vi "PH_Beamline.set GUI Refs.vi"(0 "i ref in":refnum<vi>, 1 "Class":string, 2 "PH Beamline GUI Refs":T3, 3 "PH_BL-Master GUI Refs":T2, 4 "System Information GUI Refs":T1, 5 "error in (no error)":errorcluster) -> (14 "i ref out":refnum<vi>, 19 "error out":errorcluster)   [LabVIEW 2014, in "PH_Beamline.lvlib"]
uses:
  PH_Beamline.lvlib
  PH_Beamline.GUI Refs.ctl
  PH_BL-Master/PH_BL-Master.GUI Refs.ctl
  PH_SystemInformation/PH_SystemInformation.GUI Refs.ctl
  PH_BL-Master/PH_BL-Master.lvlib
  PH_SystemInformation/PH_SystemInformation.lvlib
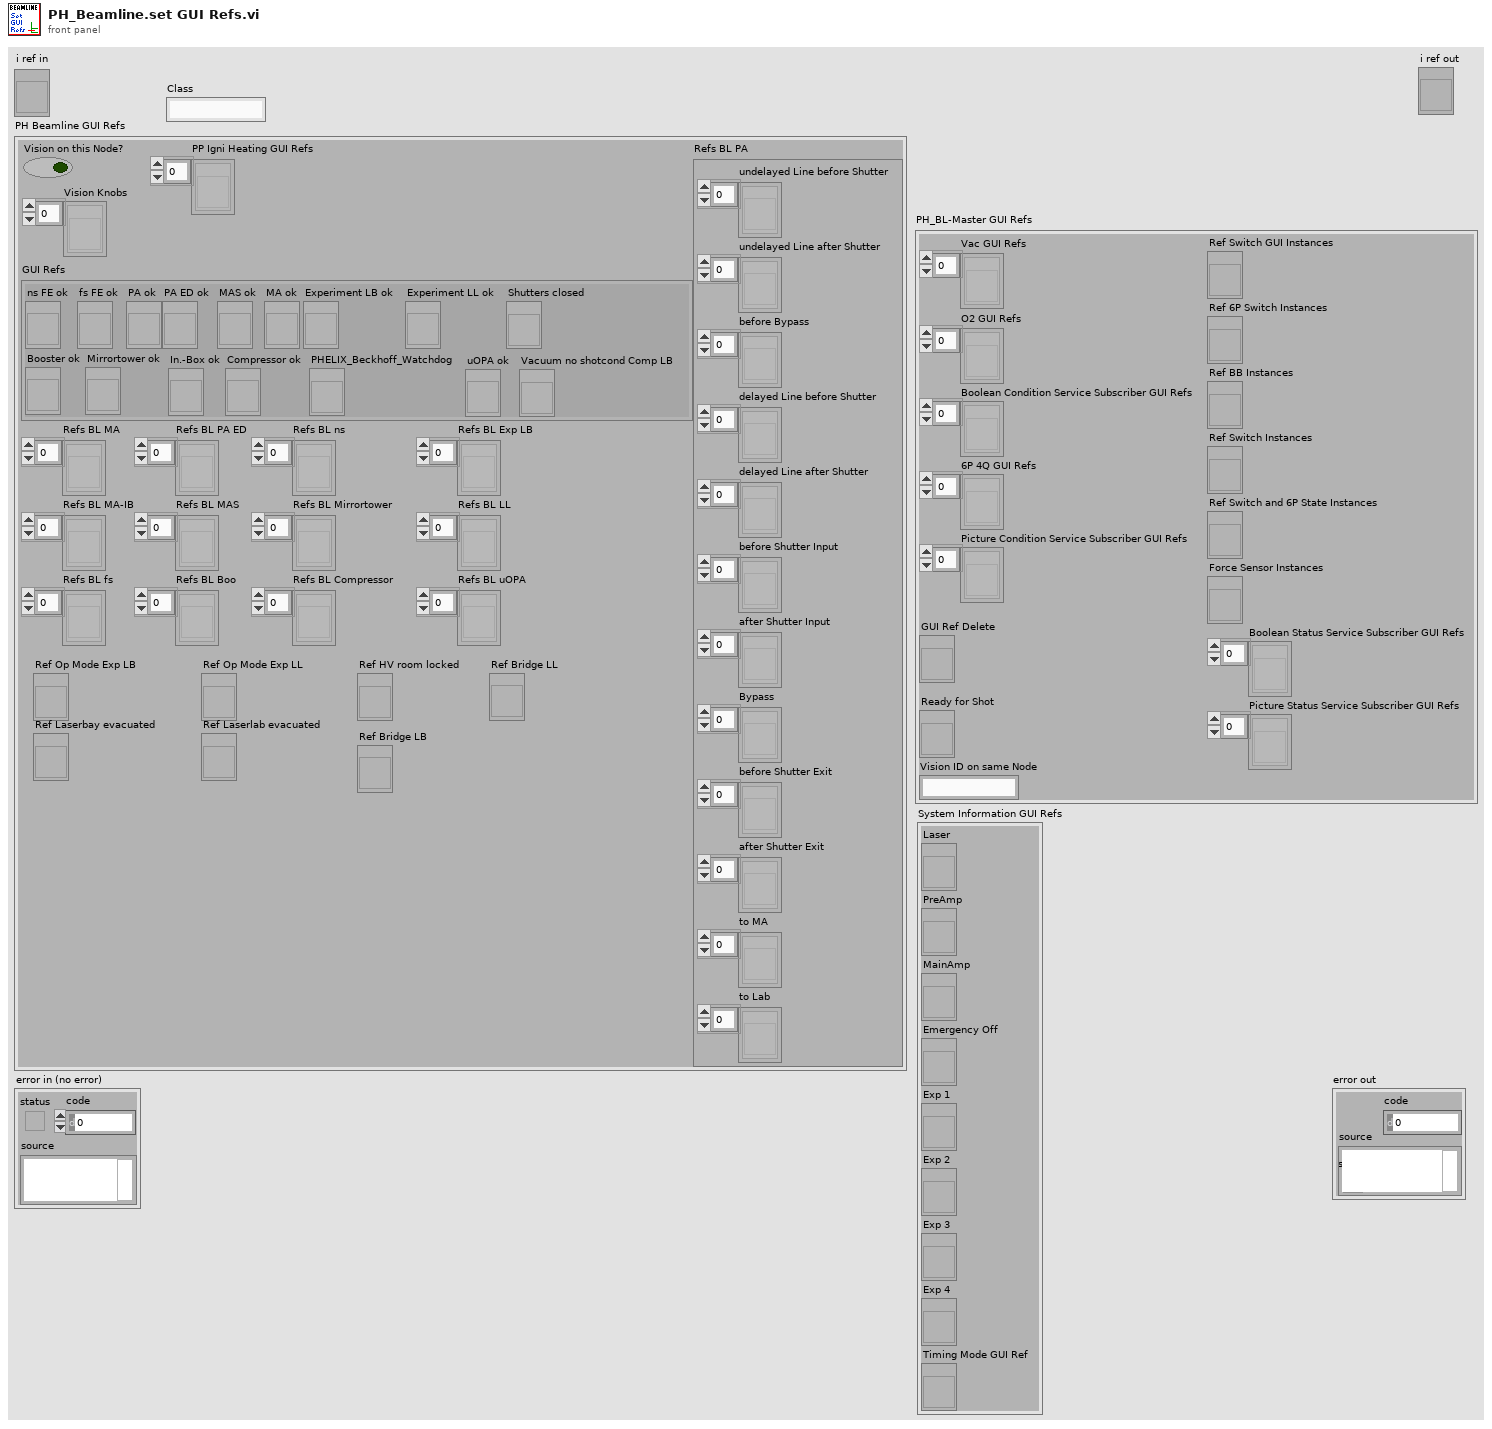
[diagram p1: front panel]
types:
  T1 = typedef "PH_SystemInformation.lvlib/PH_SystemInformation.GUI Refs.ctl" = cluster{"Laser":refnum<vi>, "PreAmp":refnum<vi>, "MainAmp":refnum<vi>, "Emergency Off":refnum<vi>, "Exp 1":refnum<vi>, "Exp 2":refnum<vi>, "Exp 3":refnum<vi>, "Exp 4":refnum<vi>, "Timing Mode GUI Ref":refnum<vi>}
  T2 = typedef "PH_BL-Master.lvlib/PH_BL-Master.GUI Refs.ctl" = cluster{"Vac GUI Refs":refnum<vi>[], "O2 GUI Refs":refnum<vi>[], "Ready for Shot":refnum<vi>, "Boolean Condition Service Subscriber GUI Refs":refnum<vi>[], "Vision ID on same Node":string, "Picture Condition Service Subscriber GUI Refs":refnum<vi>[], "6P 4Q GUI Refs":refnum<vi>[], "Ref Switch GUI Instances":refnum<vi>, "Ref 6P Switch Instances":refnum<vi>, "Ref BB Instances":refnum<vi>, "Ref Switch Instances":refnum<vi>, "Ref Switch and 6P State Instances":refnum<vi>, "Boolean Status Service Subscriber GUI Refs":refnum<vi>[], "Picture Status Service Subscriber GUI Refs":refnum<vi>[], "Force Sensor Instances":refnum<vi>, "GUI Ref Delete":refnum<vi>}
  T3 = typedef "PH_Beamline.lvlib/PH_Beamline.GUI Refs.ctl" = cluster{"Vision on this Node?":bool, "Vision Knobs":refnum<vi>[], "GUI Refs":cluster{"PA ok":refnum<vi>, "MA ok":refnum<vi>, "fs FE ok":refnum<vi>, "ns FE ok":refnum<vi>, "PA ED ok":refnum<vi>, "MAS ok":refnum<vi>, "Booster ok":refnum<vi>, "Mirrortower ok":refnum<vi>, "In.-Box ok":refnum<vi>, "Compressor ok":refnum<vi>, "Experiment LB ok":refnum<vi>, "Experiment LL ok":refnum<vi>, "PHELIX_Beckhoff_Watchdog":refnum<vi>, "Shutters closed":refnum<vi>, "uOPA ok":refnum<vi>, "Vacuum no shotcond Comp LB":refnum<vi>}, "PP Igni Heating GUI Refs":refnum<vi>[], "Refs BL PA":cluster{"undelayed Line before Shutter":refnum<vi>[], "undelayed Line after Shutter":refnum<vi>[], "before Bypass":refnum<vi>[], "delayed Line before Shutter":refnum<vi>[], "delayed Line after Shutter":refnum<vi>[], "before Shutter Input":refnum<vi>[], "after Shutter Input":refnum<vi>[], "Bypass":refnum<vi>[], "before Shutter Exit":refnum<vi>[], "after Shutter Exit":refnum<vi>[], "to MA":refnum<vi>[], "to Lab":refnum<vi>[]}, "Refs BL MA":refnum<vi>[], "Refs BL MA-IB":refnum<vi>[], "Refs BL fs":refnum<vi>[], "Refs BL PA ED":refnum<vi>[], "Refs BL MAS":refnum<vi>[], "Refs BL Boo":refnum<vi>[], "Refs BL ns":refnum<vi>[], "Refs BL Mirrortower":refnum<vi>[], "Refs BL Compressor":refnum<vi>[], "Refs BL Exp LB":refnum<vi>[], "Refs BL LL":refnum<vi>[], "Refs BL uOPA":refnum<vi>[], "Ref Op Mode Exp LB":refnum<vi>, "Ref Laserbay evacuated":refnum<vi>, "Ref Op Mode Exp LL":refnum<vi>, "Ref Laserlab evacuated":refnum<vi>, "Ref HV room locked":refnum<vi>, "Ref Bridge LB":refnum<vi>, "Ref Bridge LL":refnum<vi>}
  T4 = cluster{"undelayed Line before Shutter":refnum<vi>[], "undelayed Line after Shutter":refnum<vi>[], "before Bypass":refnum<vi>[], "delayed Line before Shutter":refnum<vi>[], "delayed Line after Shutter":refnum<vi>[], "before Shutter Input":refnum<vi>[], "after Shutter Input":refnum<vi>[], "Bypass":refnum<vi>[], "before Shutter Exit":refnum<vi>[], "after Shutter Exit":refnum<vi>[], "to MA":refnum<vi>[], "to Lab":refnum<vi>[]}
  T5 = cluster{"PA ok":refnum<vi>, "MA ok":refnum<vi>, "fs FE ok":refnum<vi>, "ns FE ok":refnum<vi>, "PA ED ok":refnum<vi>, "MAS ok":refnum<vi>, "Booster ok":refnum<vi>, "Mirrortower ok":refnum<vi>, "In.-Box ok":refnum<vi>, "Compressor ok":refnum<vi>, "Experiment LB ok":refnum<vi>, "Experiment LL ok":refnum<vi>, "PHELIX_Beckhoff_Watchdog":refnum<vi>, "Shutters closed":refnum<vi>, "uOPA ok":refnum<vi>, "Vacuum no shotcond Comp LB":refnum<vi>}
  T6 = typedef "PH_Beamline.lvlib/PH_Beamline.i attribute.ctl" = cluster{"GUI Refs":cluster{"PA ok":refnum<vi>, "MA ok":refnum<vi>, "fs FE ok":refnum<vi>, "ns FE ok":refnum<vi>, "PA ED ok":refnum<vi>, "MAS ok":refnum<vi>, "Booster ok":refnum<vi>, "Mirrortower ok":refnum<vi>, "In.-Box ok":refnum<vi>, "Compressor ok":refnum<vi>, "Experiment LB ok":refnum<vi>, "Experiment LL ok":refnum<vi>, "PHELIX_Beckhoff_Watchdog":refnum<vi>, "Shutters closed":refnum<vi>, "uOPA ok":refnum<vi>, "Vacuum no shotcond Comp LB":refnum<vi>}, "Refs BL MA":refnum<vi>[], "Refs BL MA-IB":refnum<vi>[], "Refs BL fs":refnum<vi>[], "Refs BL PA ED":refnum<vi>[], "Refs BL MAS":refnum<vi>[], "Refs BL Boo":refnum<vi>[], "Refs BL ns":refnum<vi>[], "Refs BL Mirrortower":refnum<vi>[], "Refs BL Compressor":refnum<vi>[], "Refs BL Exp LB":refnum<vi>[], "Radiation Safety":cluster{"Exp Laserbay":cluster{"Ref Op Mode":refnum<vi>, "Ref Laserbay evacuated":refnum<vi>, "Tagname LB evacuated":string, "Shot Mode":T7, "Laserbay evacuated?":i32, "Tagname HV room locked":string, "HV room locked?":i32, "Ref HV room locked":refnum<vi>, "Tagname bridged?":string, "Ref Bridge":refnum<vi>, "I<1E18W/cm²":bool}, "Exp Laserlab":cluster{"Ref Op Mode":refnum<vi>, "Ref Laserlab evacuated":refnum<vi>, "Tagname LL evacuated":string, "Shot Mode":T7, "Laserlab evacuated?":i32, "Tagname bridged?":string, "Ref Bridge":refnum<vi>, "I<1E18W/cm²":bool}}, "Refs BL LL":refnum<vi>[], "PP Igni Heating GUI Refs":refnum<vi>[], "PP Igni Heating Tagnames ":string[], "Refs BL PA":cluster{"undelayed Line before Shutter":refnum<vi>[], "undelayed Line after Shutter":refnum<vi>[], "before Bypass":refnum<vi>[], "delayed Line before Shutter":refnum<vi>[], "delayed Line after Shutter":refnum<vi>[], "before Shutter Input":refnum<vi>[], "after Shutter Input":refnum<vi>[], "Bypass":refnum<vi>[], "before Shutter Exit":refnum<vi>[], "after Shutter Exit":refnum<vi>[], "to MA":refnum<vi>[], "to Lab":refnum<vi>[]}, "BL":cluster{"YLF_BL_Status":i32, "fs_BL_Status":i32, "fs_YLF_BL_Status":i32, "ns_BL_Status":i32, "PA_Input_BL_Status":i32, "PA_UnDelay_BL_Status":i32, "PA_Delay_BL_Status":i32, "PA_BL_Status":i32, "PA_Bypass_BL_Status":i32, "PA_Exit_BL_Status":i32, "PA_LL_BL_Status":i32, "LL_BL_Status":i32, "PA_MA_BL_Status":i32, "MA_Exit_BL_Status":i32, "MA_Z6_BL_Status":i32, "Z6_BL_Status":i32, "MA_LB_BL_Status":i32, "LB_TB2_BL_Status":i32, "PA_before_Bypass_BL_Status":i32, "LB_TB3_BL_Status":i32}, "State Subsystems":cluster{"PA":bool, "MA":bool, "ns FE":bool, "fs FE":bool, "PA ED":bool, "In.-Box":bool, "MAS":bool, "Booster":bool, "Mirrortower":bool, "Compressor":bool, "Experiment LB":bool, "Experiment LL":bool, "uOPA":bool}, "Status Subscriber Information":T8, "Refs BL uOPA":refnum<vi>[], "PA_Input_2_Beam_6PWpGUI not linked?":bool, "PA_Input_Delay_6PGUI not linked?":bool, "Settings":T11}
  T7 = typedef "PH_Beamline.lvlib/PH_Beamline.Operation Mode.ctl" = i32
  T8 = typedef "PH_Beamline.lvlib/PH_Beamline.Status Subscriber Information.ctl" = cluster{"fs Swich YLF":T9, "fs Exit Shutter":T9, "ns Exit Shutter":T9, "PA Input Shutter":T9, "PA PC WP":T9, "PA PC WP 2":T9, "PA Bypass In":T9, "PA Bypass Out":T9, "PA CH 1":T9, "PA delayed":T9, "PA non delayed":T9, "PA Exit Shutter":T9, "PA Switch Lab":T9, "PA Bridge CH Input MA":T9, "MA Diffusor IB":T9, "MA IB Ready":T9, "MA CH 1":T9, "MA CH 2":T9, "MA CH 3":T9, "MA CH 4":T9, "MA Shutter Align Cam":T9, "MA Position MM5":T9, "Calorimeter Switch":T9, "BL Z6 CH 9":T9, "BL Z6 Beamdump":T9, "BL Z6 Shutter":T9, "COS Sensitivity Switch":T9, "Exp LB Shutter":T9, "Exp LB TB 2":T9, "Exp LB TB 3":T9, "PA LL Input CH":T9, "PA LL Output CH":T9, "LL Comp Input Shutter":T9, "LL Comp Output Shutter":T9, "LL Comp FF Shutter":T9, "Exp LL Shutter":T9, "MA IM In IB":T9, "MA IM Out IB":T9, "MA DB In IB":T9, "MA DB Out IB":T9, "Exp LB Shutter Interlock":T9, "Exp LL Shutter Interlock":T9, "MM1 Force Sensor":T9}
  T9 = typedef "PH_BL-Master.lvlib/PH_BL-Master.Status Subscriber Information.ctl" = cluster{"Index of element":i32, "Attributeset":T10}
  T10 = typedef "PH_BL-Master.lvlib/PH_BL-Master.Attribute Set.ctl" = enum16{"Boolean Status Service Subscriber", "Picture Status Service Subscriber"}
  T11 = typedef "PH_Beamline_Chief.lvlib/PH_Beamline_Chief.Settings.ctl" = cluster{"PA Doublepass Mode":bool, "Compressor Vaccuum LB not relevant":bool, "Windowshutter TB2 not relevant":bool, "Windowshutter TB3 not relevant":bool}
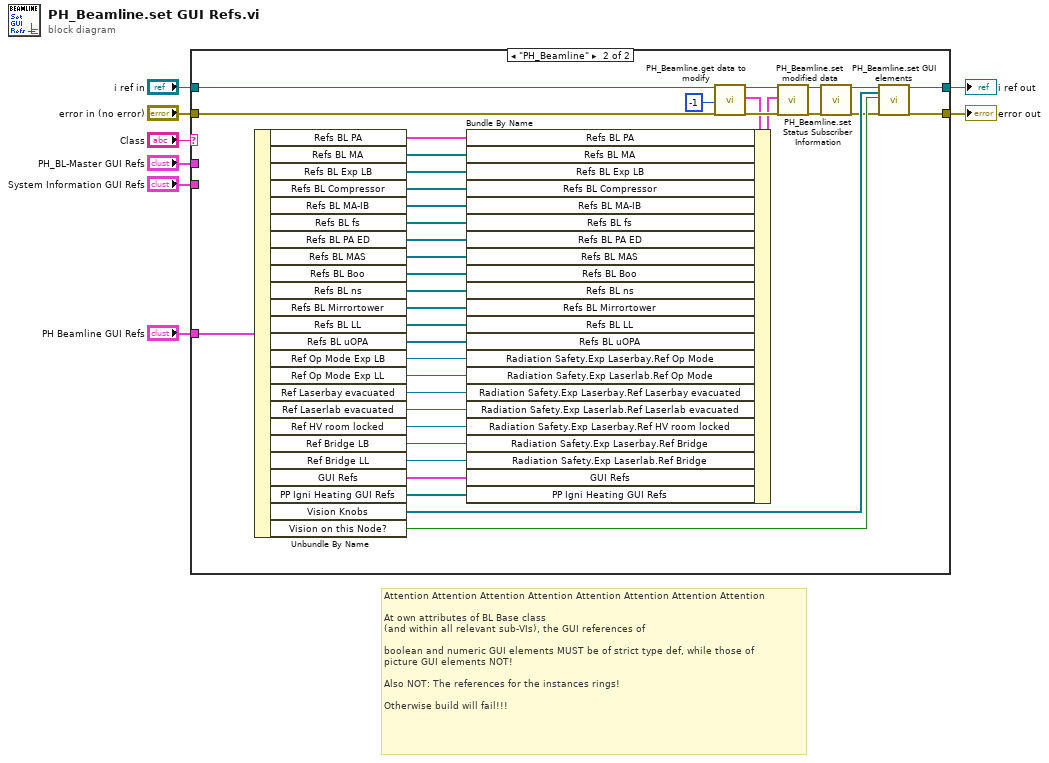
[diagram p0: block diagram]
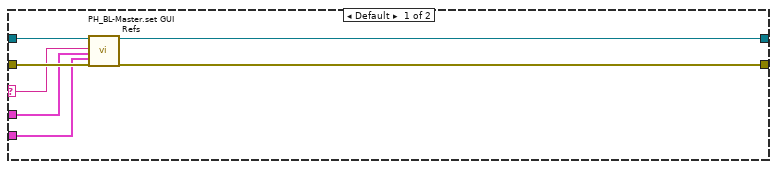
[diagram p2: hidden frame]
diagram:
  # "Attention Attention Attention Attention Attention Attention Attention Attention\n\nAt own attributes of BL Base class \n(and within all relevant sub-VIs), the GUI references of\n\nboolean and numeric GUI elements MUST be of strict type def, while those of\npicture GUI elements NOT!\n\nAlso NOT: The references for the instances rings!\n\nOtherwise build will fail!!!"
  n1 = case shown="\"PH_Beamline\"" "Class" {
    selector: "Class" -> [w11 _]
    tunnel: "i ref in" -> [w15 w53]
    tunnel: "error in (no error)" -> [w14 w52]
    tunnel: [w13 w51] -> w6
    tunnel: [w12 w50] -> w5
    tunnel: "PH Beamline GUI Refs" -> [_ w49]
    tunnel: "PH_BL-Master GUI Refs" -> [w10 _]
    tunnel: "System Information GUI Refs" -> [w9 _]
    frame Default {
      n2 = call "PH_BL-Master.set GUI Refs.vi"("i ref in"=w15, "Class"=w11, "PH_BL-Master GUI Refs"=w10, "System Information GUI Refs"=w9, "error in"=w14) -> ("i ref out"=w13:refnum<vi>, "error out"=w12:errorcluster)  [unwired: 13 in]
    }
    frame "PH_Beamline" {
      n3 = Unbundle By Name(w49) -> ("Refs BL PA"=w25:T4, "Refs BL MA"=w26:refnum<vi>[], "Refs BL Exp LB"=w27:refnum<vi>[], "Refs BL Compressor"=w28:refnum<vi>[], "Refs BL MA-IB"=w29:refnum<vi>[], "Refs BL fs"=w30:refnum<vi>[], "Refs BL PA ED"=w31:refnum<vi>[], "Refs BL MAS"=w32:refnum<vi>[], "Refs BL Boo"=w33:refnum<vi>[], "Refs BL ns"=w34:refnum<vi>[], "Refs BL Mirrortower"=w35:refnum<vi>[], "Refs BL LL"=w36:refnum<vi>[], "Refs BL uOPA"=w37:refnum<vi>[], "Ref Op Mode Exp LB"=w38:refnum<vi>, "Ref Op Mode Exp LL"=w39:refnum<vi>, "Ref Laserbay evacuated"=w40:refnum<vi>, "Ref Laserlab evacuated"=w41:refnum<vi>, "Ref HV room locked"=w42:refnum<vi>, "Ref Bridge LB"=w43:refnum<vi>, "Ref Bridge LL"=w44:refnum<vi>, "GUI Refs"=w45:T5, "PP Igni Heating GUI Refs"=w46:refnum<vi>[], "Vision Knobs"=w47:refnum<vi>[], "Vision on this Node?"=w48:bool)
      n4 = call "PH_Beamline.get data to modify.vi"("i ref in"=w53, "ms timeout (10000)"=-1, "error in (no error)"=w52) -> ("i ref out"=w24:refnum<vi>, "i attribute"=w21:T6, "error out"=w23:errorcluster)  [unwired: 13 in, 1 out]
      n5 = Bundle By Name(cluster=w21, "Refs BL PA"=w25, "Refs BL MA"=w26, "Refs BL Exp LB"=w27, "Refs BL Compressor"=w28, "Refs BL MA-IB"=w29, "Refs BL fs"=w30, "Refs BL PA ED"=w31, "Refs BL MAS"=w32, "Refs BL Boo"=w33, "Refs BL ns"=w34, "Refs BL Mirrortower"=w35, "Refs BL LL"=w36, "Refs BL uOPA"=w37, "Radiation Safety.Exp Laserbay.Ref Op Mode"=w38, "Radiation Safety.Exp Laserlab.Ref Op Mode"=w39, "Radiation Safety.Exp Laserbay.Ref Laserbay evacuated"=w40, "Radiation Safety.Exp Laserlab.Ref Laserlab evacuated"=w41, "Radiation Safety.Exp Laserbay.Ref HV room locked"=w42, "Radiation Safety.Exp Laserbay.Ref Bridge"=w43, "Radiation Safety.Exp Laserlab.Ref Bridge"=w44, "GUI Refs"=w45, "PP Igni Heating GUI Refs"=w46) -> (w20:T6)
      n6 = call "PH_Beamline.set modified data.vi"("i ref in"=w24, "i attribute"=w20, "error in (no error)"=w23) -> ("i ref out"=w19:refnum<vi>, "error out"=w17:errorcluster)  [unwired: 15 in]
      n7 = call "PH_Beamline.set Status Subscriber Information.vi"("i ref in"=w19, "error in (no error)"=w17) -> ("i ref out"=w18:refnum<vi>, "error out"=w16:errorcluster)  [unwired: 16 in]
      n8 = call "PH_Beamline.set GUI elements.vi"("i ref in"=w18, "Vision Knobs"=w47, "Vision on this node?"=w48, "error in (no error)"=w16) -> ("i ref out"=w51:refnum<vi>, "error out"=w50:errorcluster)  [unwired: 14 in]
    }
  }
  "i ref out" <- w6
  "error out" <- w5
